vi "(SubVI)_1_Pulse_gen.vi"(8 "error in":errorcluster, 11 "Line(s)":tag="Dev1/port0/line0:7") -> (0 "error out":errorcluster)   [LabVIEW 2019]
doc: "This example demonstrates how to generate digital output data using software timing.\n\nFor instructions on how to connect your signals from the DAQ device, refer to your device documentation."
uses:
  <vilib>/DAQmx/write.llb/DAQmx Write (Digital 1D Bool 1Chan 1Samp).vi
  <vilib>/DAQmx/create/channels.llb/DAQmx Create Channel (DO-Digital Output).vi
  <vilib>/DAQmx/miscellaneous.llb/DAQmx Fill In Error Info.vi
panel:
  in  "Stop":bool
  # "Channel Settings"
  # "Data to Write"
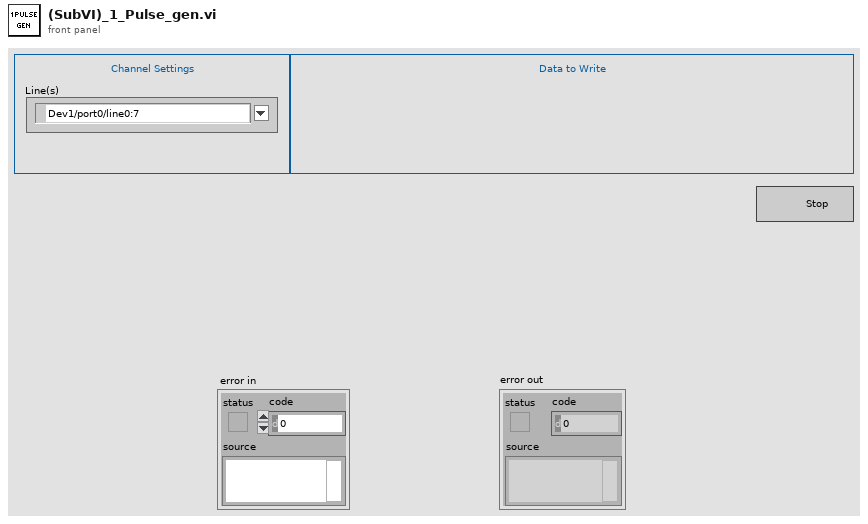
[diagram p1: front panel]
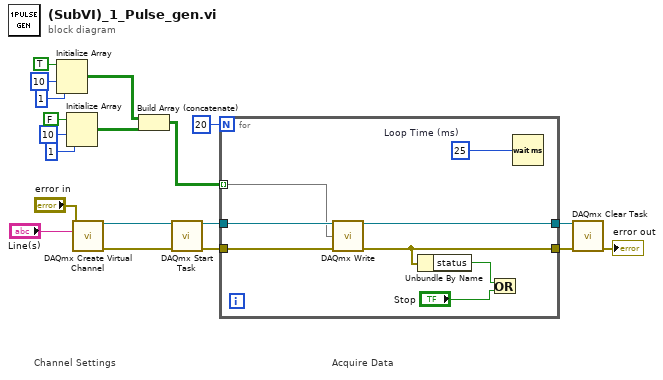
[diagram p0: block diagram]
diagram:
  # "Acquire Data"
  # "Channel Settings"
  n1 = Initialize Array(TRUE, 10 ("dimension size"), 1 ("dimension size")) -> (w6:bool[][])
  n2 = Initialize Array(FALSE, 10 ("dimension size"), 1 ("dimension size")) -> (w5:bool[][])
  n3 = call-poly <vilib>:"DAQmx Create Virtual Channel.vi"("lines"="Line(s)", "error in"="error in") -> ("task out"=w13:refnum<k21>, "error out"=w14:errorcluster)  [unwired: 12 in]
  n4 = Build Array (concatenate)(w6, w5) -> (w4:bool[][])
  n5 = call <vilib>:"DAQmx Start Task.vi"("task/channels in"=w13, "error in"=w14) -> ("task out"=w19:refnum<k21>, "error out"=w18:errorcluster)  [unwired: 12 in]
  n6 = for {
    N: 20 -> [_]
    tunnel: w19 -> [w27]
    tunnel: w18 -> [w26]
    tunnel: [w24] -> w16
    tunnel: [w25] -> w17
    tunnel: w4 -> [w20] mode=indexing
    w21 = u32 25  # Loop Time (ms)
    n7 = call-poly <vilib>:"DAQmx Write.vi"("task/channels in"=w27, "data"=w20, "error in"=w26) -> ("task out"=w25:refnum<k21>, "error out"=w24:errorcluster)  [unwired: 10 in, 1 out]
    n8 = Unbundle By Name(w24) -> ("status"=w23:bool)
    n9 = Or(x=w23, y="Stop") -> ()  [unwired: 1 out]
    n10 = Wait (ms)(milliseconds to wait=w21) -> ()  [unwired: 1 out]
  }
  n11 = call <vilib>:"DAQmx Clear Task.vi"("task in"=w17, "error in"=w16) -> ("error out"=→"error out":errorcluster)  [unwired: 13 in]
